vi "Online Status through Ping.vi"(0 "AddressToPing":string="www.google.com", 1 "Ping Method":enum16{"LongPing", "NormalPing", "FastPing"}(ring), 11 "error in (no error)":errorcluster) -> (4 "Connection?":bool, 6 "Standard Output":string, 8 "% Recieved":dbl, 10 "Average Time (ms)":dbl, 15 "error out":errorcluster)   [LabVIEW 2011]
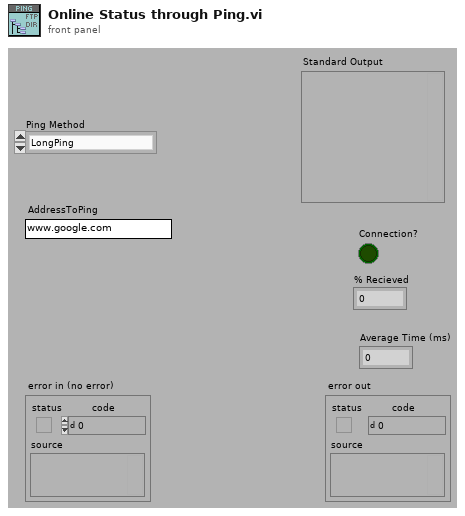
[diagram p1: front panel]
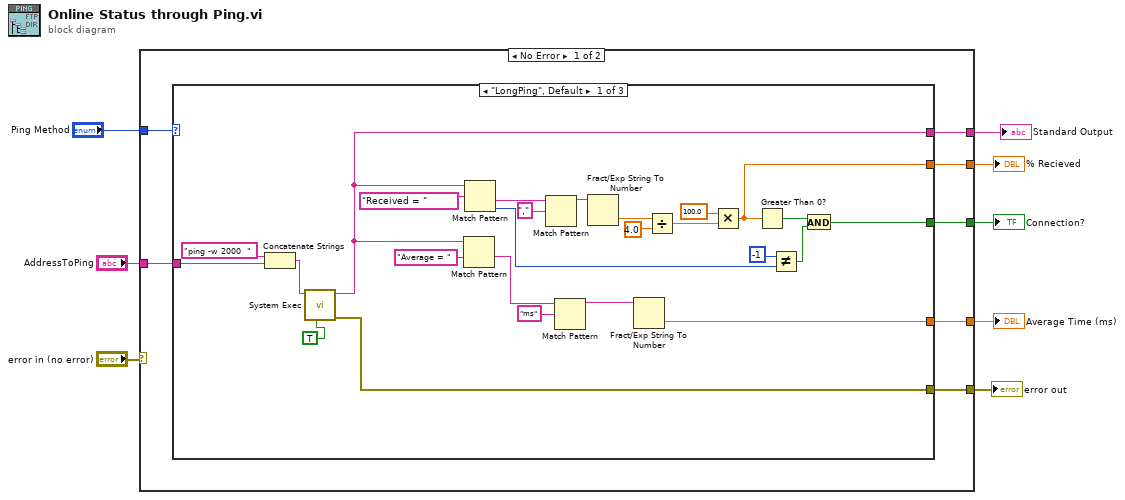
[diagram p0: block diagram]
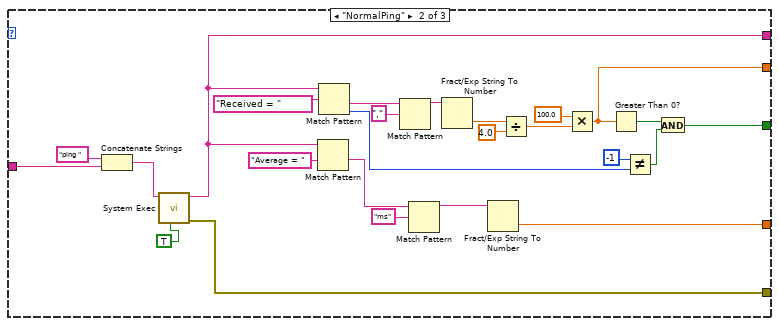
[diagram p2: hidden frame]
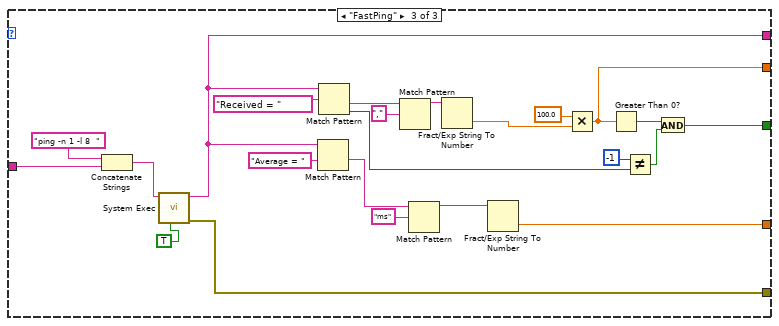
[diagram p3: hidden frame]
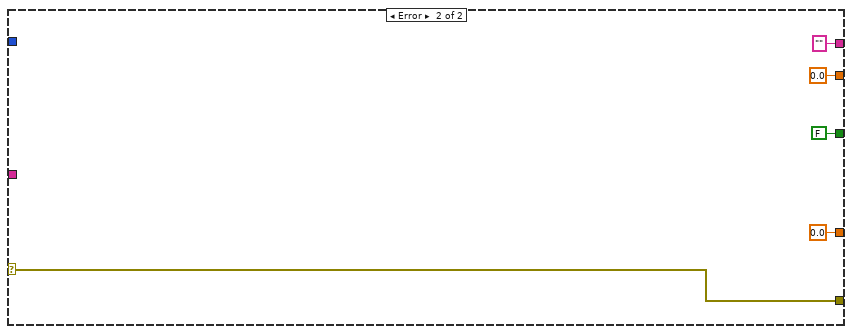
[diagram p4: hidden frame]
diagram:
  n1 = case shown="No Error" "error in (no error)" {
    selector: "error in (no error)" -> [_ w93]
    tunnel: [w15 0.0] -> w8
    tunnel: [w14 FALSE] -> w7
    tunnel: [w13 0.0] -> w6
    tunnel: [w12 w93] -> w5
    tunnel: "AddressToPing" -> [w11 _]
    tunnel: "Ping Method" -> [w10 _]
    tunnel: [w9 "" ("standard output")] -> w1
    frame No Error {
      n2 = case shown="\"LongPing\", Default" w10 {
        tunnel: [w17 w64 w87] -> w15
        tunnel: [w18 w60 w84] -> w14
        tunnel: [w19 w55 w81] -> w13
        tunnel: [w20 w45 w71] -> w12
        tunnel: w11 -> [w21 w43 w69]
        tunnel: [w16 w41 w66] -> w9
        frame "LongPing", Default {
          n3 = Concatenate Strings("ping -w 2000  ", w21) -> (w23:string)
          n4 = call <vilib>:"System Exec.vi"("run minimized? (F)"=TRUE, "command line"=w23) -> ("error out"=w20:errorcluster, "standard output"=w16:string)  [unwired: 4 in, 4 out]
          n5 = Match Pattern(string=w16, regular expression="Average = ") -> (after substring=w30:string)  [unwired: 4 out]
          n6 = Match Pattern(string=w16, regular expression="Received = ") -> (after substring=w26:string, offset past match=w38:i32)  [unwired: 3 out]
          n7 = Match Pattern(string=w26, regular expression=",") -> (before substring=w28:string)  [unwired: 4 out]
          n8 = Match Pattern(string=w30, regular expression="ms") -> (before substring=w32:string)  [unwired: 4 out]
          n9 = Fract/Exp String To Number(string=w28) -> (number=w33:dbl)  [unwired: 4 out]
          n10 = Fract/Exp String To Number(string=w32) -> (number=w19:dbl)  [unwired: 4 out]
          n11 = Divide(x=w33, y=4.0) -> (x/y=w37:dbl)
          n12 = Multiply(x=100.0, y=w37) -> (x*y=w17:dbl)
          n13 = Greater Than 0?(x=w17) -> (x > 0?=w36:bool)
          n14 = Not Equal?(x=-1, y=w38) -> (x != y?=w35:bool)
          n15 = And(x=w36, y=w35) -> (x .and. y?=w18:bool)
        }
        frame "NormalPing" {
          n16 = Concatenate Strings("ping ", w43) -> (w44:string)
          n17 = call <vilib>:"System Exec.vi"("run minimized? (F)"=TRUE, "command line"=w44) -> ("error out"=w45:errorcluster, "standard output"=w41:string)  [unwired: 4 in, 4 out]
          n18 = Match Pattern(string=w41, regular expression="Average = ") -> (after substring=w52:string)  [unwired: 4 out]
          n19 = Match Pattern(string=w41, regular expression="Received = ") -> (after substring=w48:string, offset past match=w62:i32)  [unwired: 3 out]
          n20 = Match Pattern(string=w48, regular expression=",") -> (before substring=w50:string)  [unwired: 4 out]
          n21 = Match Pattern(string=w52, regular expression="ms") -> (before substring=w54:string)  [unwired: 4 out]
          n22 = Fract/Exp String To Number(string=w50) -> (number=w56:dbl)  [unwired: 4 out]
          n23 = Fract/Exp String To Number(string=w54) -> (number=w55:dbl)  [unwired: 4 out]
          n24 = Divide(x=w56, y=4.0) -> (x/y=w61:dbl)
          n25 = Multiply(x=100.0, y=w61) -> (x*y=w64:dbl)
          n26 = Greater Than 0?(x=w64) -> (x > 0?=w59:bool)
          n27 = Not Equal?(x=-1, y=w62) -> (x != y?=w58:bool)
          n28 = And(x=w59, y=w58) -> (x .and. y?=w60:bool)
        }
        frame "FastPing" {
          n29 = Concatenate Strings("ping -n 1 -l 8  ", w69) -> (w70:string)
          n30 = call <vilib>:"System Exec.vi"("run minimized? (F)"=TRUE, "command line"=w70) -> ("error out"=w71:errorcluster, "standard output"=w66:string)  [unwired: 4 in, 4 out]
          n31 = Match Pattern(string=w66, regular expression="Average = ") -> (after substring=w78:string)  [unwired: 4 out]
          n32 = Match Pattern(string=w66, regular expression="Received = ") -> (after substring=w74:string, offset past match=w85:i32)  [unwired: 3 out]
          n33 = Match Pattern(string=w74, regular expression=",") -> (before substring=w76:string)  [unwired: 4 out]
          n34 = Match Pattern(string=w78, regular expression="ms") -> (before substring=w80:string)  [unwired: 4 out]
          n35 = Fract/Exp String To Number(string=w76) -> (number=w67:dbl)  [unwired: 4 out]
          n36 = Fract/Exp String To Number(string=w80) -> (number=w81:dbl)  [unwired: 4 out]
          n37 = Multiply(x=100.0, y=w67) -> (x*y=w87:dbl)
          n38 = Greater Than 0?(x=w87) -> (x > 0?=w83:bool)
          n39 = Not Equal?(x=-1, y=w85) -> (x != y?=w82:bool)
          n40 = And(x=w83, y=w82) -> (x .and. y?=w84:bool)
        }
      }
    }
    frame Error {
    }
  }
  "Connection?" <- w7
  "error out" <- w5
  "% Recieved" <- w8
  "Average Time (ms)" <- w6
  "Standard Output" <- w1
